vi "Test-Global.vi"() -> ()   [LabVIEW 2014]
uses:
  Terminal-Global-SetValues.vi
panel:
  in  "确定按钮":bool
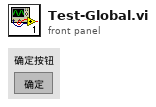
[diagram p1: front panel]
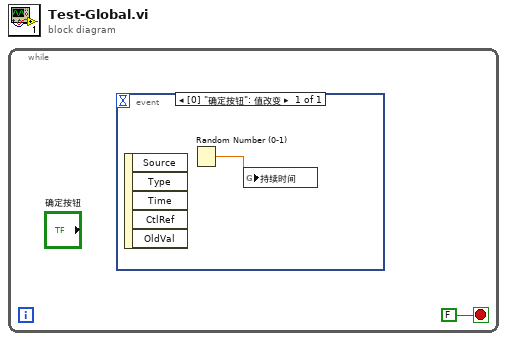
[diagram p0: block diagram]
diagram:
  n1 = while {
    stop <- FALSE stop-if-true
    n2 = event shown="[0] \"确定按钮\": 值改变" {
      selector: _ -> [_]
      dyn-events: _ -> [_]
      timeout: _ -> [_]
      event "确定按钮": Value Change {
        n3 = event-data() -> ()  [unwired: 1 in, 5 out]
        n4 = Random Number (0-1)() -> (number: 0 to 1=w2:dbl)
        n5 = global write "Terminal-Global-SetValues.vi" "持续时间"(w2) -> ()
      }
    }
  }
